vi "SeCrTs-Datalog Redundant NS creater.vi"(9 "Data FIFO Ref":T1) -> ()   [LabVIEW 2022 SP3]
uses:
  RT Controls/SeCrTs-Data FIFO.ctl
  RT Controls/SeCrTs-DiplayPC comm ctrl.ctl
  <vilib>/dex/Stream Element Allocation Mode.ctl
  SeCrTs-RT_Global_R.vi
  <resource>/objmgr/ni.dex.rc
panel:
  out "Numeric":i32
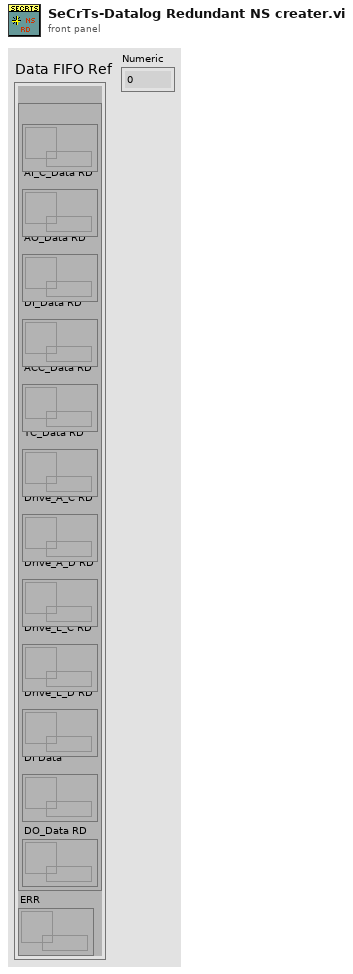
[diagram p1: front panel]
types:
  T1 = typedef "SeCrTs-Data FIFO.ctl" = cluster{"RD":cluster{"AI_V_Data RD":refnum<queue>, "AI_C_Data RD":refnum<queue>, "AO_Data RD":refnum<queue>, "DI_Data RD":refnum<queue>, "ACC_Data RD":refnum<queue>, "TC_Data RD":refnum<queue>, "Drive_A_C RD":refnum<queue>, "Drive_A_D RD":refnum<queue>, "Drive_L_C RD":refnum<queue>, "Drive_L_D RD":refnum<queue>, "DI Data":refnum<queue>, "DO_Data RD":refnum<queue>}, "ERR":refnum<queue>}
  T2 = typedef "SeCrTs-DiplayPC comm ctrl.ctl" = enum16{"Initialize", "Listen for UI Writer", "Send RT Data"}
  T3 = typedef "Stream Element Allocation Mode.ctl" = u32
  T4 = cluster{"Start DAQ":bool, "Stop DAQ":bool, "RT Stop":bool, "RT Exit":bool, "Start Seq":bool}
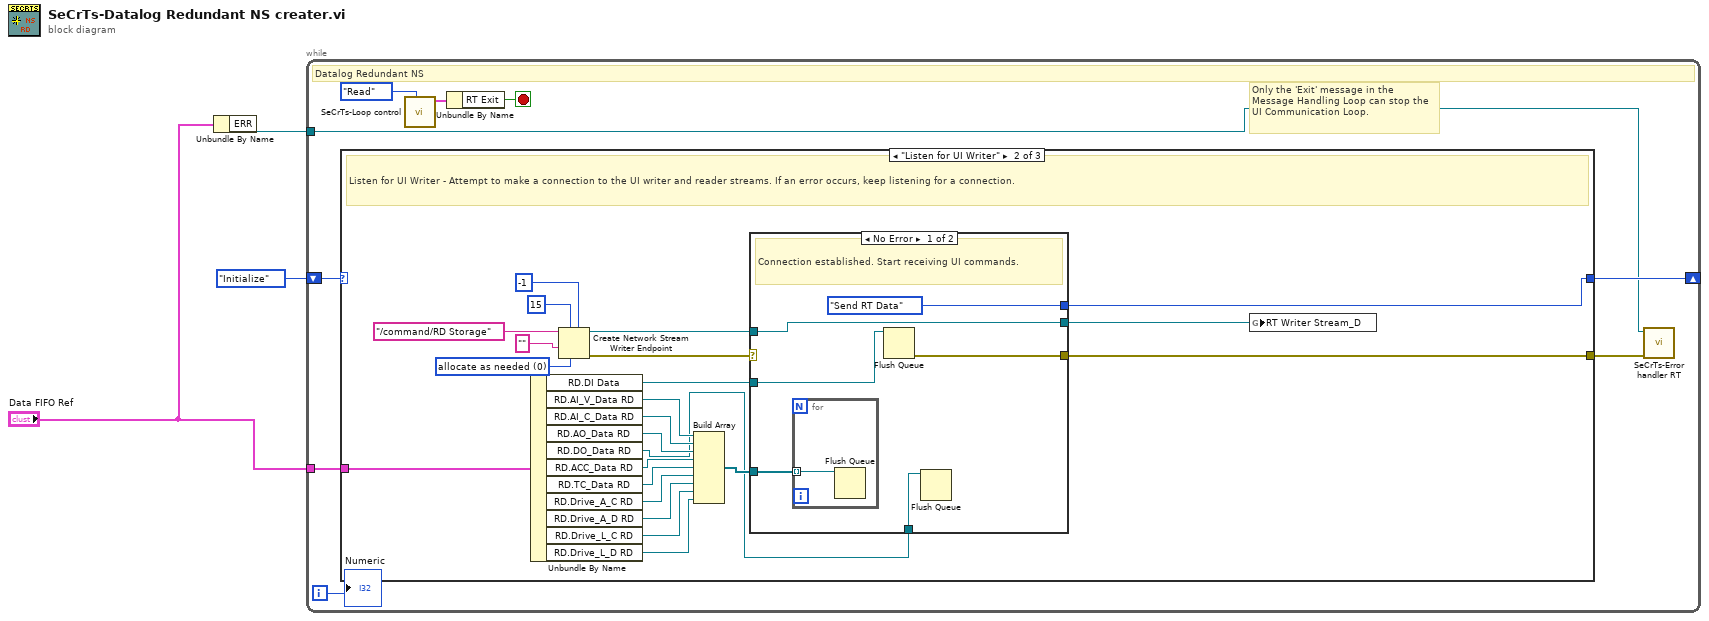
[diagram p0: block diagram]
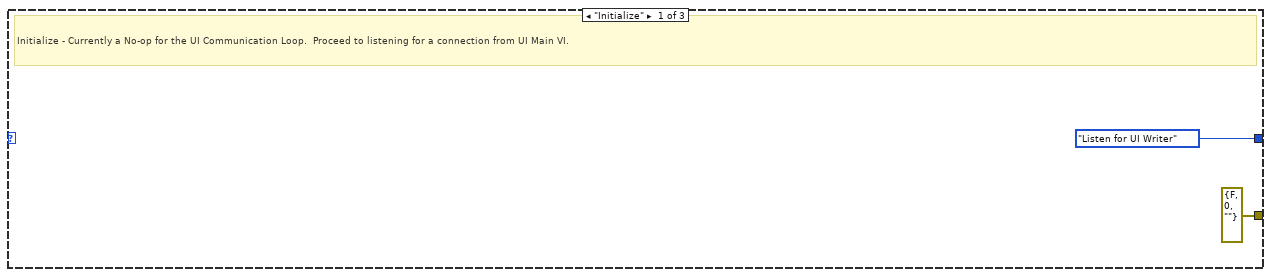
[diagram p2: hidden frame]
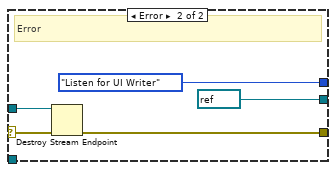
[diagram p3: hidden frame]
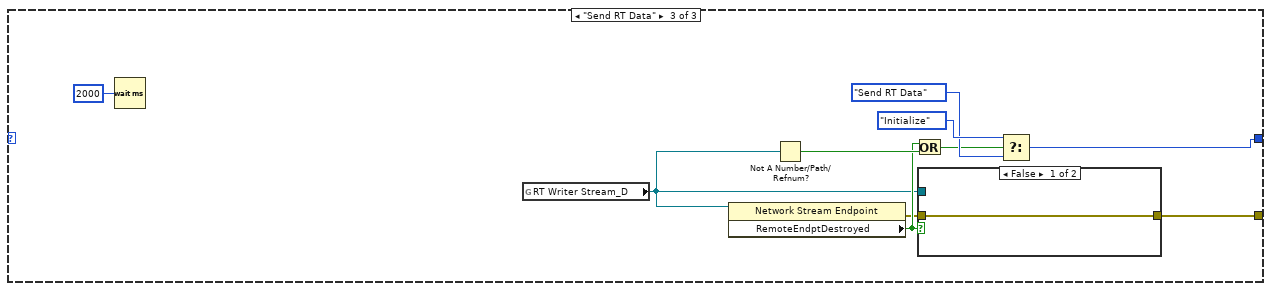
[diagram p4: hidden frame]
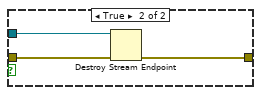
[diagram p5: hidden frame]
diagram:
  n1 = Unbundle By Name("Data FIFO Ref") -> ("ERR"=w2:refnum<queue>)
  n2 = while {
    shift-right: [w12] -> _
    shift-left: SeCrTs-DiplayPC_comm_ctrl."Initialize" -> [w11]
    tunnel: "Data FIFO Ref" -> [w10]
    tunnel: w2 -> [w6]
    i -> [w4]
    stop <- w7 stop-if-true
    # "Only the 'Exit' message in the  Message Handling Loop can stop the UI Communication Loop."
    # "Datalog Redundant NS"
    n3 = case shown="\"Listen for UI Writer\"" w11 {
      tunnel: [errorcluster {"status"=FALSE, "code"=0, "source"=""} ("error IO") w18 w50] -> w5
      tunnel: [SeCrTs-DiplayPC_comm_ctrl."Listen for UI Writer" w35 w57] -> w12
      tunnel: w10 -> [_ w32 _]
      frame "Initialize" {
        # "Initialize - Currently a No-op for the UI Communication Loop.  Proceed to listening for a connection from UI Main VI."
      }
      frame "Listen for UI Writer" {
        w15 = T3 0 items=["allocate as needed", "pre-allocate"] ("element allocation mode")
        # "Listen for UI Writer - Attempt to make a connection to the UI writer and reader streams. If an error occurs, keep listening for a connection."
        n4 = Unbundle By Name(w32) -> ("RD.DI Data"=w19:refnum<queue>, "RD.AI_V_Data RD"=w29:refnum<queue>, "RD.AI_C_Data RD"=w28:refnum<queue>, "RD.AO_Data RD"=w27:refnum<queue>, "RD.DO_Data RD"=w16:refnum<queue>, "RD.ACC_Data RD"=w26:refnum<queue>, "RD.TC_Data RD"=w25:refnum<queue>, "RD.Drive_A_C RD"=w24:refnum<queue>, "RD.Drive_A_D RD"=w23:refnum<queue>, "RD.Drive_L_C RD"=w22:refnum<queue>, "RD.Drive_L_D RD"=w21:refnum<queue>)
        n5 = Create Network Stream Writer Endpoint(5:-1 ("timeout in ms (-1)"), 6:w15, 7:15 ("writer buffer size"), 9:"" ("reader url"), 11:"/command/RD Storage" ("reader url")) -> (0:w36:errorcluster, 3:w37:refnum<k21>)  [unwired: 2 in]
        n6 = Build Array(w29, w28, w27, w26, w25, w24, w23, w22, w21) -> (w20:refnum<queue>[])
        n7 = case shown="No Error" w36 {
          selector: w36 -> [_ w47]
          tunnel: w37 -> [w40 w49]
          tunnel: [SeCrTs-DiplayPC_comm_ctrl."Send RT Data" SeCrTs-DiplayPC_comm_ctrl."Listen for UI Writer"] -> w35
          tunnel: [w40 refnum<k21> refnum ("reader url")] -> w30
          tunnel: w20 -> [w42 _]
          tunnel: w19 -> [w41 _]
          tunnel: [w39 w45] -> w18
          tunnel: w16 -> [w38 _]
          frame No Error {
            # "Connection established. Start receiving UI commands."
            n8 = for {
              tunnel: w42 -> [w44] mode=indexing
              n9 = Flush Queue(queue=w44) -> ()  [unwired: 1 in, 3 out]
            }
            n10 = Flush Queue(queue=w41) -> (error out=w39:errorcluster)  [unwired: 1 in, 2 out]
            n11 = Flush Queue(queue=w38) -> ()  [unwired: 1 in, 3 out]
          }
          frame Error {
            # "Error"
            n12 = Destroy Stream Endpoint(8:w47, 11:w49) -> (0:w45:errorcluster)
          }
        }
        n13 = global write "SeCrTs-RT_Global_R.vi" "RT Writer Stream_D"(w30) -> ()
      }
      frame "Send RT Data" {
        n14 = Wait (ms)(milliseconds to wait=u32 2000) -> ()  [unwired: 1 out]
        n15 = global read "SeCrTs-RT_Global_R.vi" "RT Writer Stream_D"() -> (w52:refnum<k21>)
        n16 = property class="Network Stream Endpoint"(reference=w52) -> (error out=w51:errorcluster, "RemoteEndptDestroyed"=w53:bool)  [unwired: 1 in, 1 out]
        n17 = Not A Number/Path/Refnum?(number/path/refnum=w52) -> (NaN/Path/Refnum?=w56:bool)
        n18 = Or(x=w53, y=w56) -> (x .or. y?=w55:bool)
        n19 = case shown="False" w53 {
          tunnel: w52 -> [_ w63]
          tunnel: w51 -> [w60 w62]
          tunnel: [w60 w61] -> w50
          frame False {
          }
          frame True {
            n20 = Destroy Stream Endpoint(8:w62, 11:w63) -> (0:w61:errorcluster)
          }
        }
        n21 = Select(t=SeCrTs-DiplayPC_comm_ctrl."Initialize", s=w55, f=SeCrTs-DiplayPC_comm_ctrl."Send RT Data") -> (s? t:f=w57:T2)
      }
    }
    n22 = call "SeCrTs-Loop control.vi"("Action"=enum16{"Init", "Write", "Read"}."Read") -> ("Loop Control out"=w9:T4)  [unwired: 9 in, 1 out]
    n23 = Unbundle By Name(w9) -> ("RT Exit"=w7:bool)
    n24 = call "SeCrTs-Error handler RT.vi"("error in"=w5, "Message Queue"=w6) -> ()  [unwired: 8 in, 2 out]
    "Numeric" <- w4
  }
